vi "Commit Scaling for Devices.vi"(0 "session in":refnum<k21>, 5 "devices":refnum<k21>="$DefaultDevices", 11 "error in (no error)":errorcluster) -> (4 "session out":refnum<k21>, 15 "error out":errorcluster)   [LabVIEW 2020, in "SLSC.lvlib"]
doc: "Commits all scaling parameters with pending changes to all physical channels that the devices contain. If you set scaling parameters multiple times between commits, this VI commits only the last value of the scaling parameters."
uses:
  <vilib>/SLSC/SLSC.lvlib
  nislsclvapi.dll
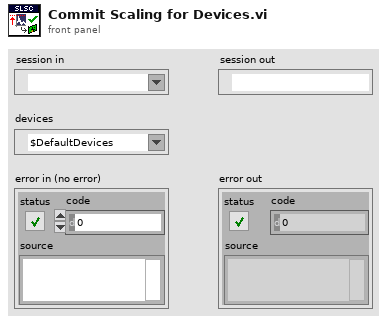
[diagram p1: front panel]
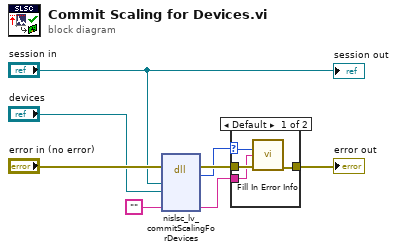
[diagram p0: block diagram]
diagram:
  n1 = dll-call lib="nislsclvapi.*" fn="nislsc_lv_commitScalingForDevices"(error in="error in (no error)", "session"="session in", "devices"="devices", "extendedErrorInfo"="") -> (error out=w6:errorcluster, "return type"=w5:i32, "extendedErrorInfo"=w7:string)  [unwired: 6 in, 1 out]
  n2 = case shown="Default" w5 {
    selector: w5 -> [w9 _]
    tunnel: w7 -> [w10 _]
    tunnel: w6 -> [w12 w13]
    tunnel: [w11 w13] -> w4
    frame Default {
      n3 = call <vilib>:"Fill In Error Info.vi"("status code"=w9, "extended error info"=w10, "error in"=w12) -> ("error out"=w11:errorcluster)  [unwired: 12 in]
    }
    frame 0 {
    }
  }
  "error out" <- w4
  "session out" <- "session in"
